vi "Example - Insert into a Table_140605.vi"() -> ()   [LabVIEW 2011]
doc: "This example opens a connection to a database specified by the Connection string (replace the DNS name with your database) inserts a new row into the table \"myOtherTable\" (replace the SQL string with your own SQL query)."
panel:
  in  "郵件編號":string
  out "error out":errorcluster
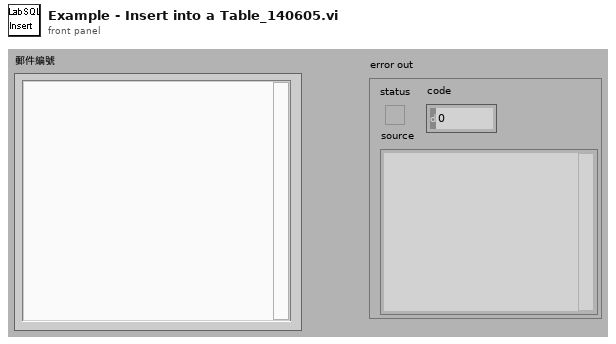
[diagram p1: front panel]
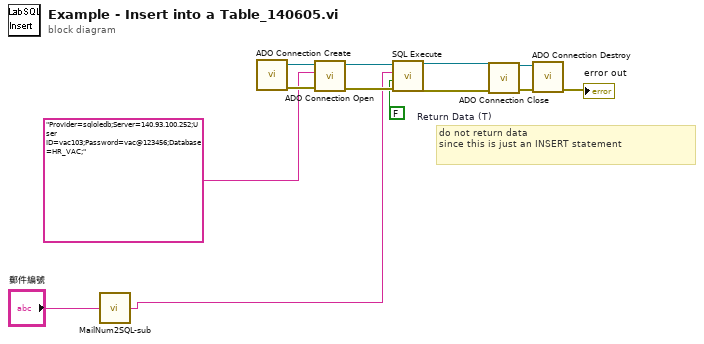
[diagram p0: block diagram]
diagram:
  w4 = FALSE  # Return Data (T)
  # "do not return data\nsince this is just an INSERT statement"
  n1 = call "MailNum2SQL-sub.vi"("mail numbers"="郵件編號") -> ("SQL String"=w1:string)
  n2 = call "ADO Connection Create.vi"() -> ("error out"=w12:errorcluster, "ADODB._Connection Out"=w13:refnum<k7>)  [unwired: 10 in]
  n3 = call "ADO Connection Open.vi"("error in (no error)"=w12, "ConnectionString"="Provider=sqloledb;Server=140.93.100.252;User ID=vac103;Password=vac@123456;Database=HR_VAC;" ("ConnectionString 2"), "ADODB._Connection In"=w13) -> ("error out"=w10:errorcluster, "ADODB._Connection Out"=w11:refnum<k7>)  [unwired: 7 in]
  n4 = call "SQL Execute.vi"("error in (no error)"=w10, "Return Data (T)"=w4, "Command Text"=w1, "ADODB._Connection In"=w11) -> ("error out"=w9:errorcluster, "ADODB._Connection Out"=w8:refnum<k7>)  [unwired: 4 in, 2 out]
  n5 = call "ADO Connection Close.vi"("error in (no error)"=w9, "ADODB._Connection In"=w8) -> ("error out"=w7:errorcluster, "ADODB._Connection Out"=w6:refnum<k7>)  [unwired: 8 in]
  n6 = call "ADO Connection Destroy.vi"("error in (no error)"=w7, "ADODB._Connection In"=w6) -> ("error out"=→"error out":errorcluster)  [unwired: 9 in]
